vi "To and From Array Test.vi"() -> (0 "error out":errorcluster, 2 "Lines Equal":bool, 3 "Class Equal":bool)   [LabVIEW 2018, in "Benchmark PID tests.lvlib"]
uses:
  Benchmark PID tests.lvlib
  module/configuration/Benchmark PID configuration.lvclass/Benchmark PID configuration.ctl
  <vilib>/NI/Tag Bus Module Framework/channel/TBM channel.lvclass
  module/configuration/Benchmark PID configuration.lvclass
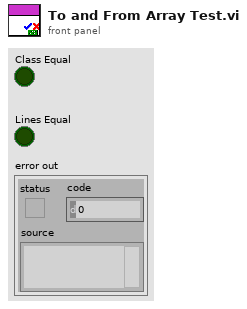
[diagram p1: front panel]
types:
  T1 = typedef "Benchmark PID configuration.lvclass/Line.ctl" = cluster{"channel":refnum<class "TBM channel.lvclass">}
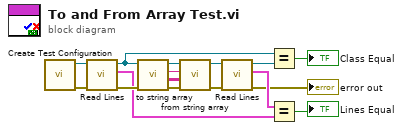
[diagram p0: block diagram]
diagram:
  n1 = call "Create Test Configuration.vi"() -> ("error out"=w8:errorcluster, "Module Configuration"=w9:refnum<class "Benchmark PID configuration.lvclass">)  [unwired: 6 in, 4 out]
  n2 = call "Read Lines.vi"("error in (no error)"=w8, "Benchmark PID configuration in"=w9) -> ("error out"=w10:errorcluster, "Lines"=w4:T1[], "Benchmark PID configuration out"=w6:refnum<class "Benchmark PID configuration.lvclass">)  [unwired: 7 in]
  n3 = call-dynamic "to string array.vi"("error in (no error)"=w10, "Benchmark PID configuration in"=w6) -> ("error out"=w16:errorcluster, "Array"=w15:string[][], "version"=w14:string, "Benchmark PID configuration out"=w13:refnum<class "Benchmark PID configuration.lvclass">)  [unwired: 6 in]
  n4 = call-dynamic "from string array.vi"("error in (no error)"=w16, "String Array"=w15, "version"=w14, "Benchmark PID configuration in"=w13) -> ("error out"=w11:errorcluster, "Benchmark PID configuration out"=w12:refnum<class "Benchmark PID configuration.lvclass">)  [unwired: 6 in]
  n5 = call "Read Lines.vi"("error in (no error)"=w11, "Benchmark PID configuration in"=w12) -> ("error out"=→"error out":errorcluster, "Lines"=w5:T1[], "Benchmark PID configuration out"=w7:refnum<class "Benchmark PID configuration.lvclass">)  [unwired: 7 in]
  n6 = Equal?(x=w6, y=w7) -> (x = y?=→"Class Equal":bool)
  n7 = Equal?(x=w5, y=w4) -> (x = y?=→"Lines Equal":bool)
